vi "Create ToolStrip Seperator.vi"(8 "error in (no error)":errorcluster caption="错误输入（无错误）") -> (0 "error out":errorcluster caption="错误输出", 2 "ItemRef":refnum<k24>, 3 "ToolsStripSeperator 输出":refnum<class "ToolsStripSeperator.lvclass"> caption="DNL_LabVIEW Object out")   [LabVIEW 2013, in "ToolsStripSeperator.lvclass"]
uses:
  ToolsStripSeperator.lvclass
  System.Windows.Forms
  ToolsStripSeperator.lvclass/ToolsStripSeperator.ctl
panel:
  in  "ToolsStripSeperator 输入":refnum<class "ToolsStripSeperator.lvclass"> caption="DNL_LabVIEW Object in"
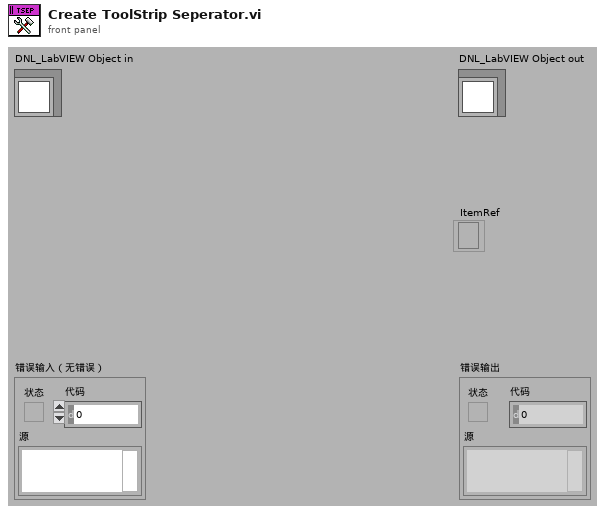
[diagram p1: front panel]
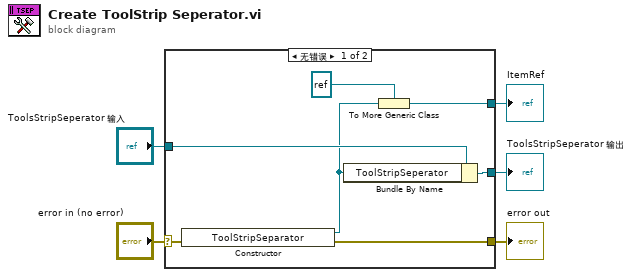
[diagram p0: block diagram]
diagram:
  n1 = case shown="无错误" "error in (no error)" {
    selector: "error in (no error)" -> [w10 w14]
    tunnel: [w6 w14] -> w4
    tunnel: [w11 w13] -> w2
    tunnel: "ToolsStripSeperator 输入" -> [w12 w13]
    tunnel: [w7 _] -> w1
    frame No Error {
      n2 = constructor class="ToolStripSeparator"(error in=w10) -> (reference out=w9:refnum<k24>, error out=w6:errorcluster)  [unwired: 2 in, 1 out]
      n3 = Bundle By Name(cluster=w12, "ToolStripSeperator"=w9) -> (w11:refnum<class "ToolsStripSeperator.lvclass">)
      n4 = To More Generic Class(target class=refnum<k24> refnum ("value"), reference=w9) -> (generic class reference=w7:refnum<k24>)
    }
    frame Error {
    }
  }
  "error out" <- w4
  "ToolsStripSeperator 输出" <- w2
  "ItemRef" <- w1
